vi "setStage.vi"(8 "error in (no error)":errorcluster, 11 "ActionEditor in":refnum<class "ActionEditor.lvclass">) -> (0 "error out":errorcluster, 3 "ActionEditor out":refnum<class "ActionEditor.lvclass">)   [LabVIEW 2011, in "Views.lvlib" / "ScriptEditor.lvlib" / "ActionEditor.lvclass"]
uses:
  ActionEditor.lvclass
  ActionEditor.lvclass/ActionEditor.ctl
  Tools/Scripting/ScriptingEvent/ScriptEvent.lvclass
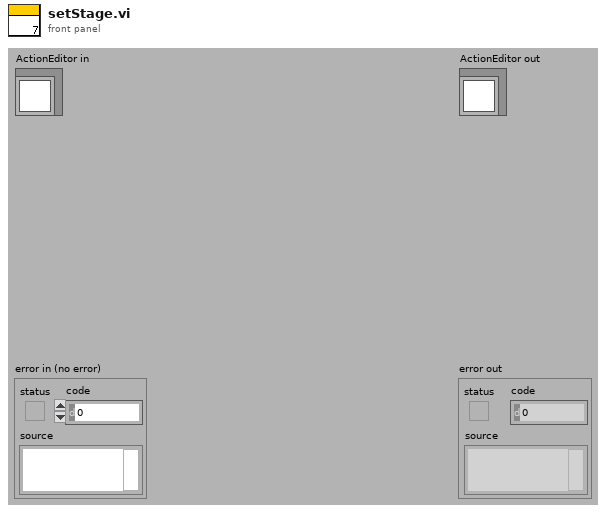
[diagram p1: front panel]
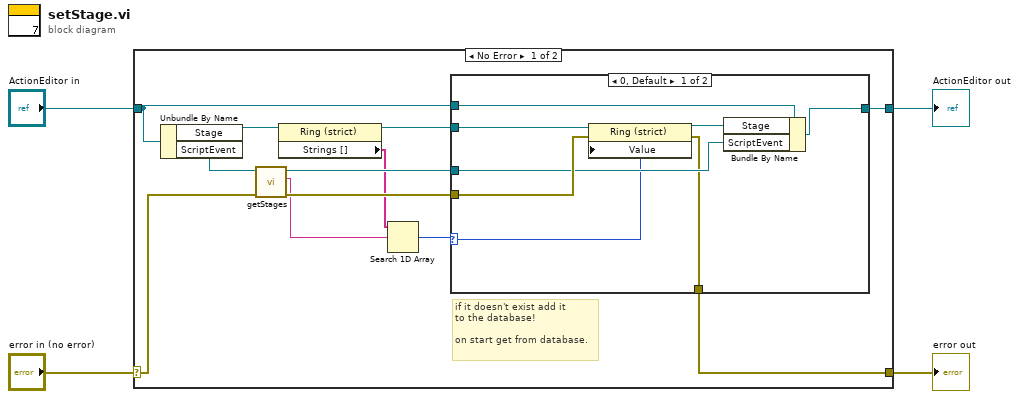
[diagram p0: block diagram]
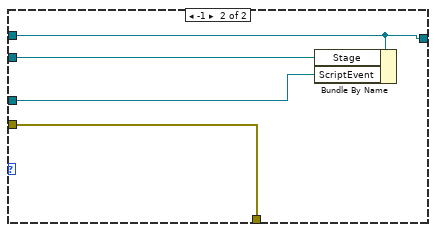
[diagram p2: hidden frame]
diagram:
  n1 = case shown="No Error" "error in (no error)" {
    selector: "error in (no error)" -> [w15 w30]
    tunnel: [w9 w30] -> w3
    tunnel: [w11 w29] -> w1
    tunnel: "ActionEditor in" -> [w12 w29]
    frame No Error {
      # "if it doesn't exist add it\nto the database!\n\non start get from database."
      n2 = Unbundle By Name(w12) -> ("Stage"=w14:refnum<vi>, "ScriptEvent"=w16:refnum<class "ScriptEvent.lvclass">)
      n3 = call "getStages.vi"("error in (no error)"=w15, "ScriptEvent.lvclass in"=w16) -> ("error out"=w13:errorcluster, "Stage"=w6:string, "ScriptEvent.lvclass out"=w10:refnum<class "ScriptEvent.lvclass">)  [unwired: 7 in]
      n4 = property class="Ring (strict)"(reference=w14) -> (reference out=w8:refnum<vi>, "Strings []"=w7:string[])  [unwired: 1 in, 1 out]
      n5 = Search 1D Array(1D array=w7, element=w6) -> (index of element=w5:i32)  [unwired: 1 in]
      n6 = case shown="0, Default" w5 {
        selector: w5 -> [w17 _]
        tunnel: w13 -> [w24 w25]
        tunnel: w12 -> [w22 w28]
        tunnel: [w21 w28] -> w11
        tunnel: w10 -> [w20 w26]
        tunnel: [w19 w25] -> w9
        tunnel: w8 -> [w18 w27]
        frame 0, Default {
          n7 = property class="Ring (strict)"(reference=w18, error in=w24, "Value"=w17) -> (reference out=w23:refnum<vi>, error out=w19:errorcluster)
          n8 = Bundle By Name(cluster=w22, "Stage"=w23, "ScriptEvent"=w20) -> (w21:refnum<class "ActionEditor.lvclass">)
        }
        frame -1 {
          n9 = Bundle By Name(cluster=w28, "Stage"=w27, "ScriptEvent"=w26) -> ()  [unwired: 1 out]
        }
      }
    }
    frame Error {
    }
  }
  "error out" <- w3
  "ActionEditor out" <- w1
